vi "cSM Optimize Error Source.vi"(6 "Previous State":string, 8 "Error in":errorcluster) -> (0 "Error out":errorcluster)   [LabVIEW 2021, in "EDT VIE.lvlib"]
uses:
  EDT VIE.lvlib
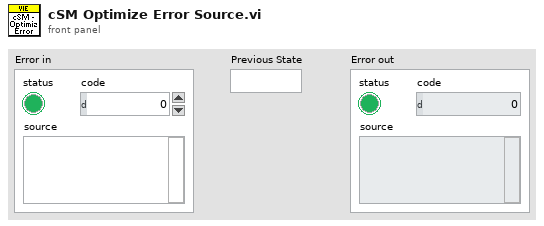
[diagram p1: front panel]
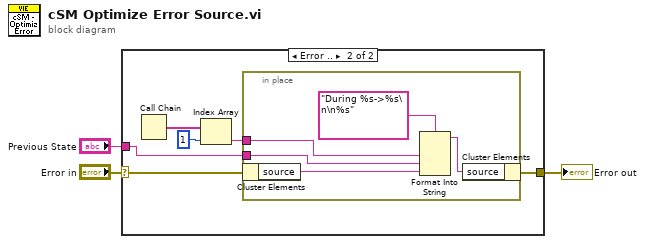
[diagram p0: block diagram]
diagram:
  n1 = case shown="Error .." "Error in" {
    selector: "Error in" -> [w4 w8]
    tunnel: [w4 w7] -> w2
    tunnel: "Previous State" -> [_ w5]
    frame No Error {
    }
    frame Error {
      n2 = Call Chain() -> (call chain=w10:string[])
      n3 = Index Array(array=w10, index=1) -> (element=w6:string)
      n4 = in-place {
        in-place-border: w6 -> [w14]
        in-place-border: w5 -> [w13]
        n5 = in-place-cluster #1(w8) -> ("source"=w11:string)
        n6 = Format Into String(format string="During %s->%s\n\n%s", w14, w13, w11) -> (resulting string=w12:string)  [unwired: 2 in, 1 out]
        n7 = in-place-cluster #1("source"=w12) -> (w7:errorcluster)
      }
    }
  }
  "Error out" <- w2
